vi "Select Grey.vi"(8 "error in (no error)":errorcluster, 10 "Coords":T1, 11 "ColorSelector in":refnum<class "ColorSelector.lvclass">) -> (0 "error out":errorcluster, 3 "ColorSelector out":refnum<class "ColorSelector.lvclass">)   [LabVIEW 2015, in "ColorSelector.lvclass"]
doc: "Select Grey determines the selected grey from the Grey Selector.\n<b> </b> <b> </b>\n©2017 Q Software Innovations, LLC (QSI)\nwritten by Quentin Alldredge\nproduced in LabVIEW 2015\n\nsupport@qsoftwareinnovations.com\nwww.qsoftwareinnovations.com\n\nAll rights reserved.\n\nRedistribution and use in source and binary forms, with or without modification, are permitted provided that the following conditions are met:\n\n * Redistributions of source code must retain the above copyright notice, this list of conditions and the following disclaimer.\n * Redistributions in binary form must reproduce the above copyright notice, this list of conditions and the following disclaimer in the documentation and/or other materials provided with the distribution.\n * Neither the name of Q Software Innovations, LLC. nor the names of its contributors may be used to endorse or promote products derived from this software without specific prior written permission.\n\nTHIS SOFTWARE IS PROVIDED BY THE COPYRIGHT HOLDERS AND CONTRIBUTORS \"AS IS\" AND ANY EXPRESS OR IMPLIED WARRANTIES, INCLUDING, BUT NOT LIMITED TO, THE IMPLIED WARRANTIES OF MERCHANTABILITY AND FITNESS FOR A PARTICULAR PURPOSE ARE DISCLAIMED. IN NO EVENT SHALL THE COPYRIGHT OWNER OR CONTRIBUTORS BE LIABLE FOR ANY DIRECT, INDIRECT, INCIDENTAL, SPECIAL, EXEMPLARY, OR CONSEQUENTIAL DAMAGES (INCLUDING, BUT NOT LIMITED TO, PROCUREMENT OF SUBSTITUTE GOODS OR SERVICES; LOSS OF USE, DATA, OR PROFITS; OR BUSINESS INTERRUPTION) HOWEVER CAUSED AND ON ANY THEORY OF LIABILITY, WHETHER IN CONTRACT, STRICT LIABILITY, OR TORT (INCLUDING NEGLIGENCE OR OTHERWISE) ARISING IN ANY WAY OUT OF THE USE OF THIS SOFTWARE, EVEN IF ADVISED OF THE POSSIBILITY OF SUCH DAMAGE."
uses:
  ColorSelector.lvclass
  <vilib>/Utility/miscctls.llb/LVPoint32TypeDef.ctl
  ColorSelector.lvclass/ColorSelector.ctl
  Read GreySelectPic.vi
  Write GreyGridCoords.vi
  Read ColorGridCoords.vi
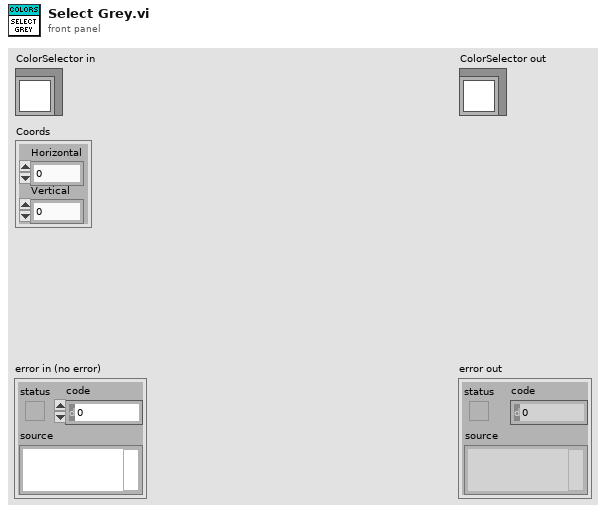
[diagram p1: front panel]
types:
  T1 = typedef "LVPoint32TypeDef.ctl" = cluster{"Horizontal":i32, "Vertical":i32}
  T2 = typedef "imagedata.ctl" = cluster{"image type":i32, "image depth":i32, "image":u8[], "mask":u8[], "colors":u32[], "Rectangle":cluster{"left":i16, "top":i16, "right":i16, "bottom":i16}}
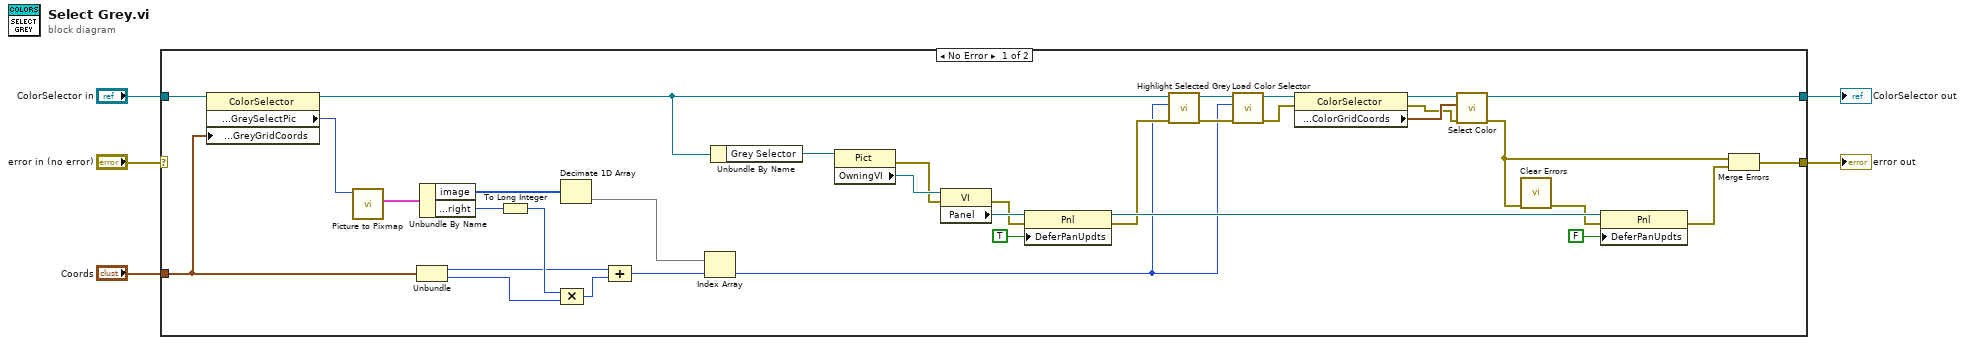
[diagram p0: block diagram]
diagram:
  n1 = case shown="No Error" "error in (no error)" {
    selector: "error in (no error)" -> [_ w42]
    tunnel: [w13 w42] -> w4
    tunnel: [w27 w41] -> w2
    tunnel: "ColorSelector in" -> [w29 w41]
    tunnel: "Coords" -> [w7 _]
    frame No Error {
      n2 = property class="ColorSelector"(reference=w29, "State Data:Accessors:GreyGridCoords"=w7) -> (reference out=w9:refnum<class "ColorSelector.lvclass">, "State Data:Accessors:GreySelectPic"=w32:picture)  [unwired: 1 in, 1 out]
      n3 = call <vilib>:"Picture to Pixmap.vi"("picture"=w32) -> ("image data"=w39:T2)  [unwired: 9 in, 1 out]
      n4 = Unbundle(w7) -> ("Horizontal"=w36:i32, "Vertical"=w8:i32)
      n5 = Unbundle By Name(w39) -> ("image"=w35:u8[], "Rectangle.right"=w31:i16)
      n6 = To Long Integer(number=w31) -> (32bit integer=w38:i32)
      n7 = Decimate 1D Array(w35) -> (w34:u8[])  [unwired: 2 out]
      n8 = Compound Arithmetic op=MULTIPLY(w38, w8) -> (w37:i32)
      n9 = Compound Arithmetic op=ADD(w36, w37) -> (w33:i32)
      n10 = Index Array(array=w34, index=w33) -> (element=w6:u8)
      n11 = Unbundle By Name(w9) -> ("Grey Selector"=w40:refnum<vi>)
      n12 = property class="Pict"(reference=w40) -> (error out=w22:errorcluster, "OwningVI"=w23:refnum<vi>)  [unwired: 1 in, 1 out]
      n13 = property class="VI"(reference=w23, error in=w22) -> (error out=w20:errorcluster, "Panel"=w21:refnum<vi>)  [unwired: 1 out]
      n14 = property class="Pnl"(reference=w21, error in=w20, "DeferPanUpdts"=TRUE ("Defer Panel Updates")) -> (reference out=w15:refnum<vi>, error out=w14:errorcluster)
      n15 = call "Highlight Selected Grey.vi"("error in (no error)"=w14, "Grayscale Index (0-255)"=w6, "ColorSelector in"=w9) -> ("error out"=w24:errorcluster, "ColorSelector (dup)"=w30:refnum<class "ColorSelector.lvclass">)  [unwired: 7 in]
      n16 = call "Load Color Selector.vi"("error in (no error)"=w24, "Grayscale Index (0-255)"=w6, "ColorSelector in"=w30) -> ("error out"=w18:errorcluster, "ColorSelector out"=w28:refnum<class "ColorSelector.lvclass">)  [unwired: 7 in]
      n17 = property class="ColorSelector"(reference=w28, error in=w18) -> (reference out=w26:refnum<class "ColorSelector.lvclass">, error out=w17:errorcluster, "State Data:Accessors:ColorGridCoords"=w25:T1)
      n18 = call "Select Color.vi"("error in (no error)"=w17, "Coords in"=w25, "ColorSelector in"=w26) -> ("error out"=w12:errorcluster, "ColorSelector (dup)"=w27:refnum<class "ColorSelector.lvclass">)  [unwired: 7 in]
      n19 = call <vilib>:"Clear Errors.vi"("error in (no error)"=w12) -> ("error out"=w11:errorcluster)  [unwired: 5 in, 1 out]
      n20 = property class="Pnl"(reference=w15, error in=w11, "DeferPanUpdts"=FALSE ("Defer Panel Updates")) -> (error out=w10:errorcluster)  [unwired: 1 out]
      n21 = Merge Errors(w12, w10) -> (w13:errorcluster)
    }
    frame Error {
    }
  }
  "error out" <- w4
  "ColorSelector out" <- w2
